vi "APC_9049_checkAI.vi"(1 "AIdata [bar]":dbl[][](array[numeric])=array8x7200[57600 elements]) -> (0 "x = y?":bool)   [LabVIEW 2020]
doc: "This example demonstrates the procedure required to apply different NI-DAQmx Custom Scales to each virtual channel in a task. A DAQmx Task Property Node (Functions >> NI Measurements >> DAQmx - Data Acquisition >> DAQmx Advanced Task Options) is used to obtain the task's virtual channels. A DAQmx Channel Property Node (Functions >> NI Measurements >> DAQmx - Data Acquisition) is then used to set the custom scale for each virtual channel in the task.\n\nThe \"DAQmx Create Scale\" VI creates a custom scale for each channel in the channel list. *Note, make sure your Minimum and Maximum channel parameters are consistent with the range the scale will create."
panel:
  out "AI size":i32[](array[numeric])
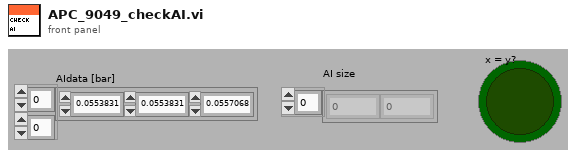
[diagram p1: front panel]
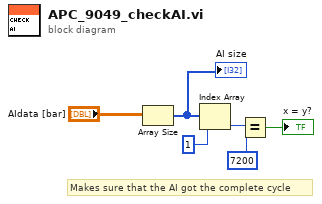
[diagram p0: block diagram]
diagram:
  # "Makes sure that the AI got the complete cycle"
  n1 = Array Size(array="AIdata [bar]") -> (size(s)=w2:i32[])
  "AI size" <- w2
  n2 = Index Array(array=w2, index=1) -> (element=w4:i32)
  n3 = Equal?(x=w4, y=7200) -> (x = y?=→"x = y?":bool)
